vi "Enter Password.vi"(8 "Error In":errorcluster) -> (0 "Error Out":errorcluster, 3 "Password Out":string)   [LabVIEW 2021]
panel:
  in  "OK":bool
  in  "Password":string
  # "Enter the Administrator Password"
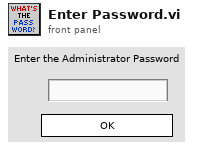
[diagram p1: front panel]
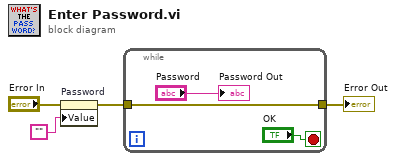
[diagram p0: block diagram]
diagram:
  n1 = property on="Password" class="Str"(error in="Error In", "Value"="") -> (error out=w3:errorcluster)  [unwired: 1 in, 1 out]
  n2 = while {
    tunnel: w3 -> [w5]
    tunnel: [w5] -> w4
    stop <- "OK" stop-if-true
    "Password Out" <- "Password"
  }
  "Error Out" <- w4
